vi "move-and-measure_NI_v1.vi"(1 "XY-in":dbl[](array[numeric]), 2 "bar-note":u8, 7 "stage-refs":T1, 11 "stage-error-in":errorcluster, 12 "counter-in":dbl format="%#_13g", 13 "meas#":dbl) -> (3 "measured-point out":dbl[](array[numeric]), 4 "logfile-line-out":string, 6 "iCorr-out":dbl, 14 "counter-out":dbl, 15 "stage-error-out":errorcluster)   [LabVIEW 2024]
uses:
  C:/Users/hpDIRC/Desktop/eic_dirc_daq-LabVIEW_new/Thorlabs.MotionControl.IntegratedStepperMotorsCLI.dll
  Thorlabs.MotionControl.IntegratedStepperMotorsCLI.dll
  C:/Users/hpDIRC/Desktop/eic_dirc_daq-LabVIEW_new/Thorlabs.MotionControl.Benchtop.StepperMotorCLI.dll
  Thorlabs.MotionControl.Benchtop.StepperMotorCLI.dll
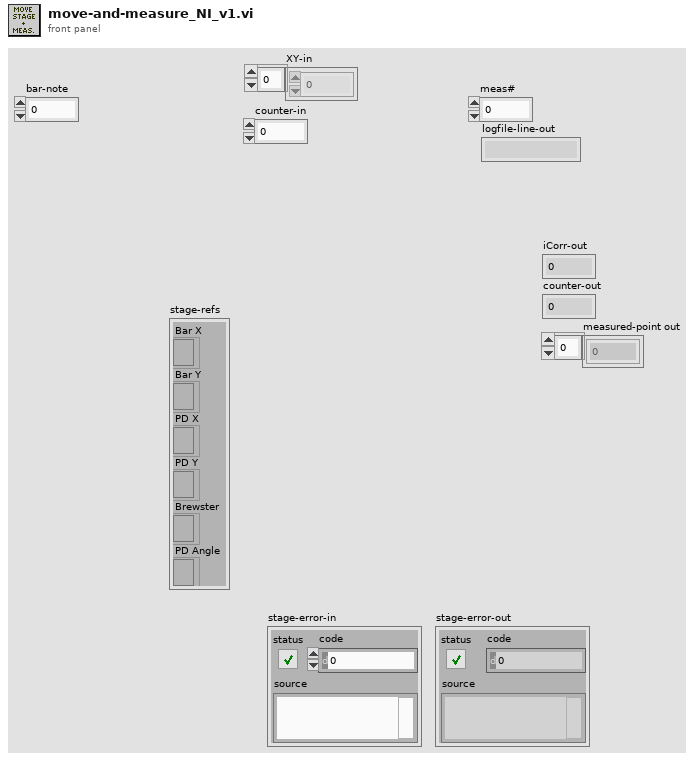
[diagram p1: front panel]
types:
  T1 = cluster{"Bar X":refnum<k24>, "Bar Y":refnum<k24>, "PD X":refnum<k24>, "PD Y":refnum<k24>, "Brewster":refnum<k24>, "PD Angle":refnum<k24>}
  T2 = cluster{"Bar X":dbl, "Bar Y":dbl, "PD X":dbl, "PD Y":dbl, "BMA":dbl, "PDA":dbl}
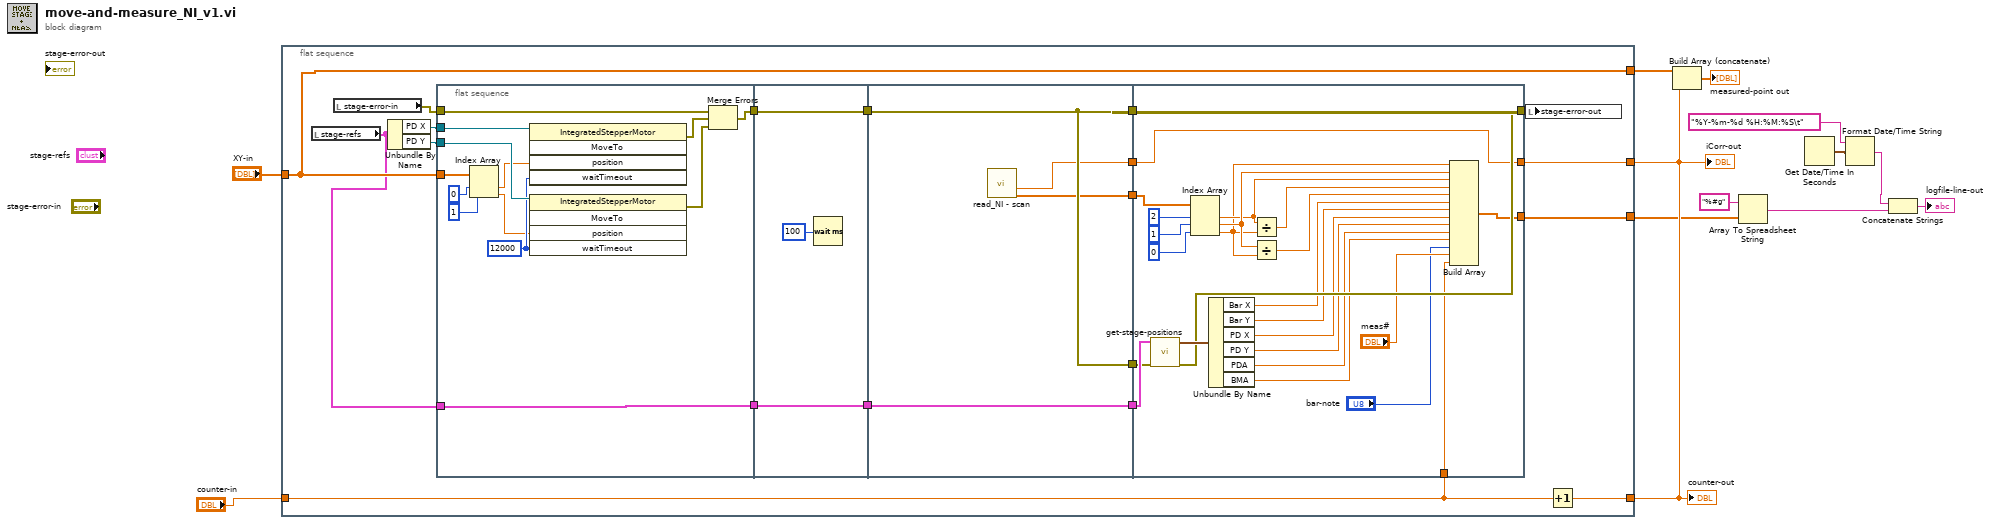
[diagram p0: block diagram]
diagram:
  n1 = flat-sequence {
    tunnel: [w30] -> w9
    tunnel: "XY-in" -> [w27]
    tunnel: "counter-in" -> [w19]
    tunnel: [w20] -> w8
    tunnel: [w27] -> w10
    tunnel: [w18] -> w5
    frame #0 {
      n2 = local read "stage-refs"() -> (w22:T1)
      n3 = local read "stage-error-in"() -> (w28:errorcluster)
      n4 = Unbundle By Name(w22) -> ("PD X"=w32:refnum<k24>, "PD Y"=w31:refnum<k24>)
      n5 = flat-sequence {
        tunnel: w32 -> [w43]
        tunnel: w31 -> [w42]
        tunnel: w28 -> [w36]
        tunnel: w27 -> [w34]
        tunnel: [w35] -> w17
        tunnel: [w33] -> w15
        tunnel: w22 -> [w33]
        tunnel: w17 -> [w48]
        tunnel: [w48] -> w16
        tunnel: w15 -> [w47]
        tunnel: [w47] -> w14
        tunnel: w16 -> [w51]
        tunnel: [w49] -> w26
        tunnel: [w51] -> w25
        tunnel: [w50] -> w24
        tunnel: [w52] -> w23
        tunnel: w14 -> [w52]
        tunnel: [w51] -> w21
        tunnel: [w67] -> w29
        tunnel: [w56] -> w30
        tunnel: w26 -> [w56]
        tunnel: w25 -> [_]
        tunnel: w24 -> [w73]
        tunnel: w23 -> [w69]
        tunnel: w21 -> [w68]
        tunnel: w19 -> [w60]
        tunnel: [w58] -> w18
        frame #0 {
          w41 = 12000 ("waitTimeout")
          n6 = Index Array(array=w34, index #1=0 ("index"), index #2=1 ("index")) -> (element #1=w38:dbl, element #2=w37:dbl)
          n7 = invoke class="IntegratedStepperMotor" method="MoveTo"(reference=w43, "position"=w38, "waitTimeout"=w41) -> (error out=w45:errorcluster)  [unwired: 2 in, 4 out]
          n8 = invoke class="IntegratedStepperMotor" method="MoveTo"(reference=w42, "position"=w37, "waitTimeout"=w41) -> (error out=w44:errorcluster)  [unwired: 2 in, 4 out]
          n9 = Merge Errors(w36, w45, w44) -> (w35:errorcluster)
        }
        frame #1 {
          n10 = Wait (ms)(milliseconds to wait=u32 100) -> ()  [unwired: 1 out]
        }
        frame #2 {
          n11 = call "read_NI - scan.vi"() -> ("all_pds"=w50:dbl[], "-pd3/pd1"=w49:dbl)  [unwired: 8 in, 2 out]
        }
        frame #3 {
          n12 = call "get-stage-positions.vi"("error in (no error)"=w68, "Cluster"=w69) -> ("error out"=w67:errorcluster, "stage positions"=w70:T2)  [unwired: 8 in]
          n13 = Index Array(array=w73, index #1=2 ("index"), index #2=1 ("index"), index #3=0 ("index")) -> (element #1=w55:dbl, element #2=w57:dbl, element #3=w53:dbl)
          n14 = Unbundle By Name(w70) -> ("Bar X"=w66:dbl, "Bar Y"=w65:dbl, "PD X"=w64:dbl, "PD Y"=w63:dbl, "PDA"=w62:dbl, "BMA"=w61:dbl)
          n15 = Divide(x=w55, y=w53) -> (x/y=w72:dbl)
          n16 = Divide(x=w57, y=w53) -> (x/y=w71:dbl)
          n17 = Build Array(w53, w57, w55, w72, w71, w66, w65, w64, w63, w62, w61, "bar-note", "meas#", w60) -> (w58:dbl[])
        }
      }
      n18 = local write "stage-error-out"(w29) -> ()
      n19 = Increment(x=w19) -> (x+1=w20:dbl)
    }
  }
  n20 = Build Array (concatenate)(w10, w9, w8) -> (→"measured-point out":dbl[])
  n21 = Array To Spreadsheet String(array=w5, 3:"%#g" ("format string")) -> (spreadsheet string=w3:string)  [unwired: 1 in]
  n22 = Get Date/Time In Seconds() -> (seconds since 1Jan1904=w7:timestamp)
  n23 = Format Date/Time String(time format string (%c)="%Y-%m-%d %H:%M:%S\t", seconds (now)=w7) -> (date/time string=w2:string)  [unwired: 1 in]
  n24 = Concatenate Strings(w2, w3) -> (→"logfile-line-out":string)
  "iCorr-out" <- w9
  "counter-out" <- w8
